vi "v_sizematrix.vi"(1 "xyz":dbl[](array[numeric])=[1.0, 1.0, 1.0]) -> (0 "matrix":dbl[][](array[numeric])=[[1.0, 0.0, 0.0, 0.0], [0.0, 1.0, 0.0, 0.0], [0.0, 0.0, 1.0, 0.0], [0.0, 0.0, 0.0, 1.0]])   [LabVIEW 2011]
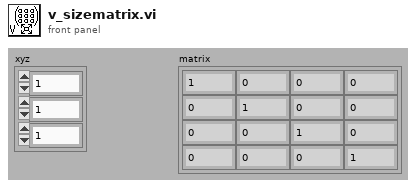
[diagram p1: front panel]
types:
  T1 = cluster{"xyz[0]":dbl, "xyz[1]":dbl, "xyz[2]":dbl}
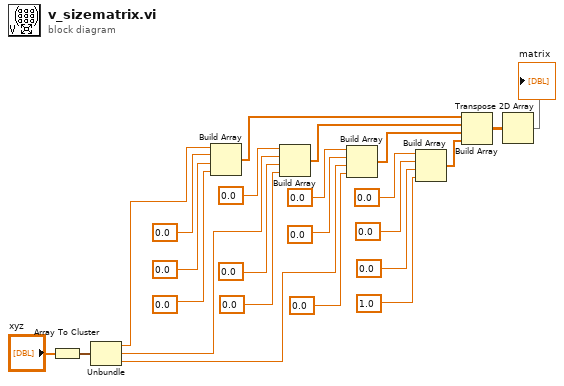
[diagram p0: block diagram]
diagram:
  n1 = Array To Cluster(array="xyz") -> (cluster=w7:T1)
  n2 = Unbundle(w7) -> ("xyz[0]"=w5:dbl, "xyz[1]"=w6:dbl, "xyz[2]"=w4:dbl)
  n3 = Build Array(w5, 0.0, 0.0, 0.0) -> (w11:dbl[])
  n4 = Build Array(0.0, w6, 0.0, 0.0) -> (w10:dbl[])
  n5 = Build Array(0.0, 0.0, w4, 0.0) -> (w9:dbl[])
  n6 = Build Array(0.0, 0.0, 0.0, 1.0) -> (w14:dbl[])
  n7 = Build Array(w11, w10, w9, w14) -> (w21:dbl[][])
  n8 = Transpose 2D Array(2D array=w21) -> (transposed array=→"matrix":dbl[][])
